vi "Terminate.vi"(8 "error in (no error)":errorcluster, 10 "Message in":refnum<class "TerminateMessage.lvclass">, 11 "Tomo in":refnum<class "Tomo.lvclass">) -> (0 "error out":errorcluster, 3 "Tomo out":refnum<class "Tomo.lvclass">)   [LabVIEW 2012, in "Tomo.lvclass"]
doc: "This member function is called when the statemachine in the run.vi receives an 'terminate' command. It closes the RabbitMQ connection. \n\nOverride this member function in your derived class to release all previously acquired resources (but don't forget to call the parent method). If your component has subcomponents, they count as resources, and you have to release them by calling their own terminate functions."
uses:
  Tomo.lvclass
  <vilib>/Distrio/Murmex/TerminateMessage/TerminateMessage.lvclass
  <vilib>/Distrio/Murmex/Murmex/Murmex.lvclass
  Tomo.lvclass/Tomo.ctl
panel:
  # "This method is called when the TERMINATE\ntrigger is sent. \n\nOverride this method when your component needs to\nrespond to this trigger. \n\nCall parent for proper implementation"
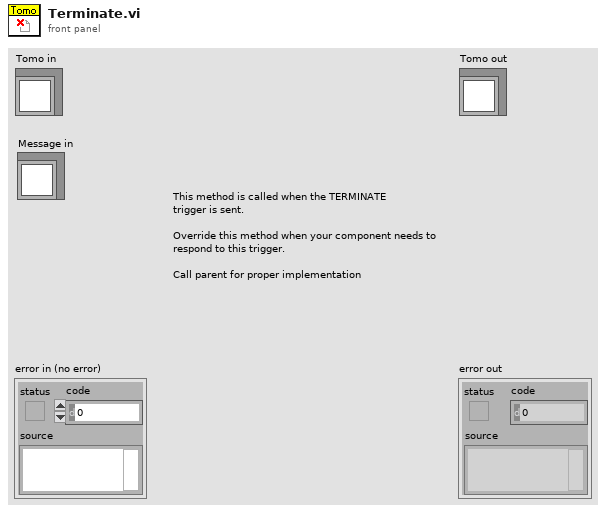
[diagram p1: front panel]
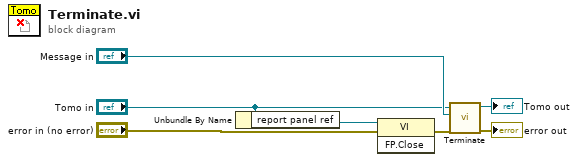
[diagram p0: block diagram]
diagram:
  n1 = Unbundle By Name("Tomo in") -> ("report panel ref"=w4:refnum<vi>)
  n2 = invoke class="VI" method="FP.Close"(reference=w4, error in="error in (no error)") -> (error out=w3:errorcluster)  [unwired: 1 in, 2 out]
  n3 = call-parent "Terminate.vi"("error in (no error)"=w3, "Message in"="Message in", "Murmex in"="Tomo in") -> ("error out"=→"error out":errorcluster, "Murmex out"=→"Tomo out":refnum<class "Tomo.lvclass">)  [unwired: 7 in]
